vi "Framework.Load Transfer Groups.vi"(8 "error in (no error)":errorcluster, 11 "Framework in":refnum<class "Framework.lvclass">) -> (0 "error out":errorcluster, 2 "Transfer Groups":refnum<class "Transfer Group.lvclass">[](array[class]), 3 "Framework out":refnum<class "Framework.lvclass">)   [LabVIEW 2017, in "DSF Core.lvlib" / "Framework.lvclass"]
uses:
  Framework.lvclass
  Transfer/Transfer Group.lvclass
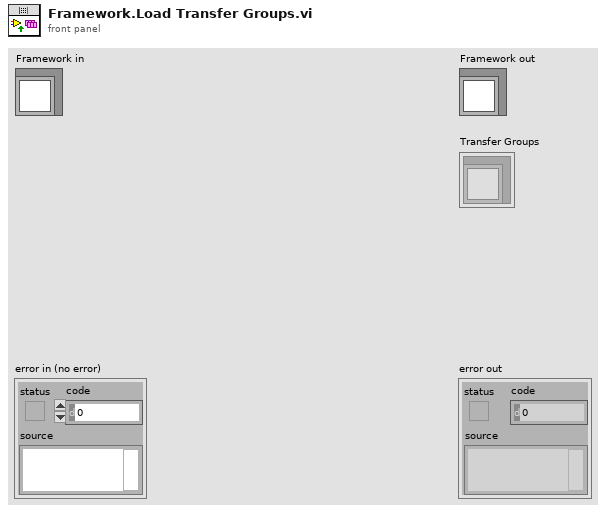
[diagram p1: front panel]
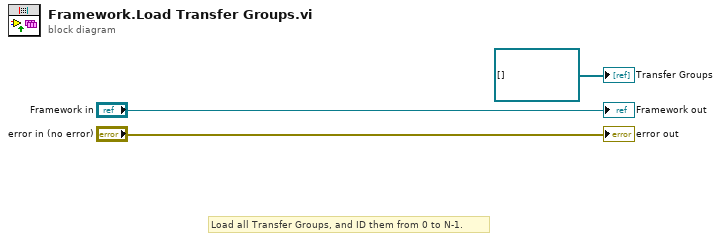
[diagram p0: block diagram]
diagram:
  # "Load all Transfer Groups, and ID them from 0 to N-1."
  "error out" <- "error in (no error)"
  "Framework out" <- "Framework in"
  "Transfer Groups" <- refnum<class "Transfer Group.lvclass">[] [] ("Transfers")
